vi "FPGA_AI ADC Loop.vi"(10 "AI ADC IO":T1={"AI_A"={"CONV"="RMC/DIO0", "RST"="RMC/DIO64", "SCK"="RMC/DIO17", "CS"="RMC/DIO81", "BUSY"="RMC/DIO16", "DOUT_A"="RMC/DIO48", "DOUT_B"="RMC/DIO80", "t_RST (ticks)"=0, "t_CONV (ticks)"=0, "t_BUSYMAX (ticks)"=0}, "AI_B"={"CONV"="RMC/DIO33", "RST"="RMC/DIO18", "SCK"="RMC/DIO50", "CS"="RMC/DIO32", "BUSY"="RMC/DIO65", "DOUT_A"="RMC/DIO49", "DOUT_B"="RMC/DIO82", "t_RST (ticks)"=0, "t_CONV (ticks)"=0, "t_BUSYMAX (ticks)"=0}, "AI_C"={"CONV"="RMC/DIO51", "RST"="RMC/DIO84", "SCK"="RMC/DIO2", "CS"="RMC/DIO66", "BUSY"="RMC/DIO19", "DOUT_A"="RMC/DIO83", "DOUT_B"="RMC/DIO1", "t_RST (ticks)"=0, "t_CONV (ticks)"=0, "t_BUSYMAX (ticks)"=0}}, 11 "AI ADC Loop Data In":T2={"AI ADC Loop State"=enum."Initialize", "AI Data"=[0, 0, 0, 0, 0, 0, 0, 0, 0, 0, 0, 0, 0, 0, 0, 0, 0, 0, 0, 0, 0, 0, 0, 0]}) -> (3 "AI ADC Loop Data Out":T2={"AI ADC Loop State"=enum."Initialize", "AI Data"=[0, 0, 0, 0, 0, 0, 0, 0, 0, 0, 0, 0, 0, 0, 0, 0, 0, 0, 0, 0, 0, 0, 0, 0]})   [LabVIEW 2018]
uses:
  Data Def/FPGA_AI ADC Loop Data.ctl
  Data Def/FPGA_AI ADC Loop State.ctl
  Data Def/FPGA_AI ADC IO.ctl
  24AIO/AI/AI_FPGA.lvlib
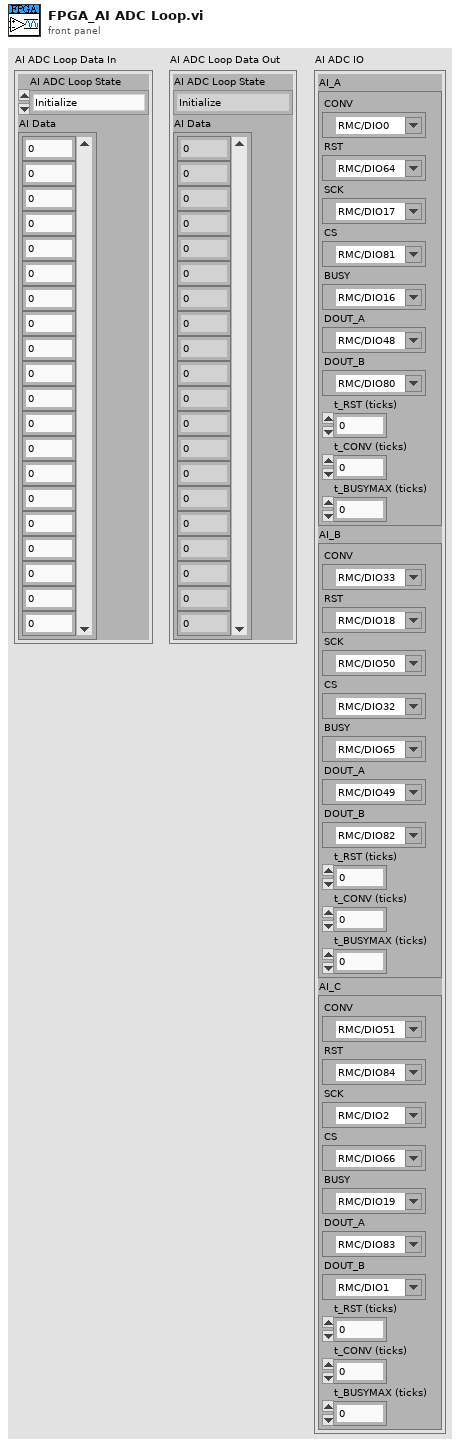
[diagram p1: front panel]
types:
  T1 = typedef "FPGA_AI ADC IO.ctl" = cluster{"AI_A":cluster{"CONV":refnum<k21>, "RST":refnum<k21>, "SCK":refnum<k21>, "CS":refnum<k21>, "BUSY":refnum<k21>, "DOUT_A":refnum<k21>, "DOUT_B":refnum<k21>, "t_RST (ticks)":u32, "t_CONV (ticks)":u32, "t_BUSYMAX (ticks)":u32}, "AI_B":cluster{"CONV":refnum<k21>, "RST":refnum<k21>, "SCK":refnum<k21>, "CS":refnum<k21>, "BUSY":refnum<k21>, "DOUT_A":refnum<k21>, "DOUT_B":refnum<k21>, "t_RST (ticks)":u32, "t_CONV (ticks)":u32, "t_BUSYMAX (ticks)":u32}, "AI_C":cluster{"CONV":refnum<k21>, "RST":refnum<k21>, "SCK":refnum<k21>, "CS":refnum<k21>, "BUSY":refnum<k21>, "DOUT_A":refnum<k21>, "DOUT_B":refnum<k21>, "t_RST (ticks)":u32, "t_CONV (ticks)":u32, "t_BUSYMAX (ticks)":u32}}
  T2 = typedef "FPGA_AI ADC Loop Data.ctl" = cluster{"AI ADC Loop State":T3, "AI Data":i16[]}
  T3 = typedef "FPGA_AI ADC Loop State.ctl" = enum16{"Initialize", "Get Data"}
  T4 = cluster{"CONV":refnum<k21>, "RST":refnum<k21>, "SCK":refnum<k21>, "CS":refnum<k21>, "BUSY":refnum<k21>, "DOUT_A":refnum<k21>, "DOUT_B":refnum<k21>, "t_RST (ticks)":u32, "t_CONV (ticks)":u32, "t_BUSYMAX (ticks)":u32}
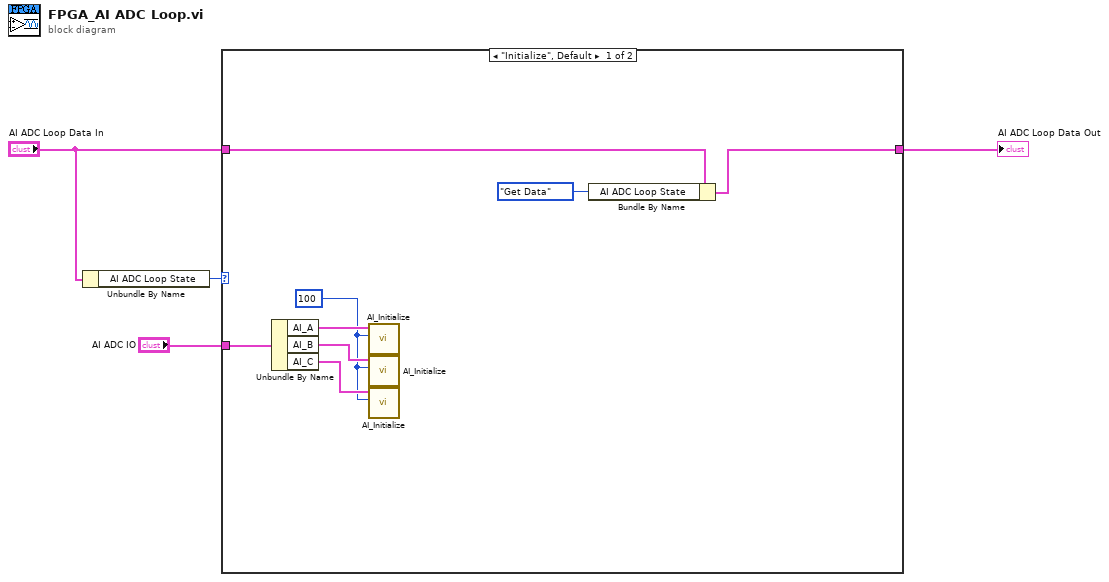
[diagram p0: block diagram]
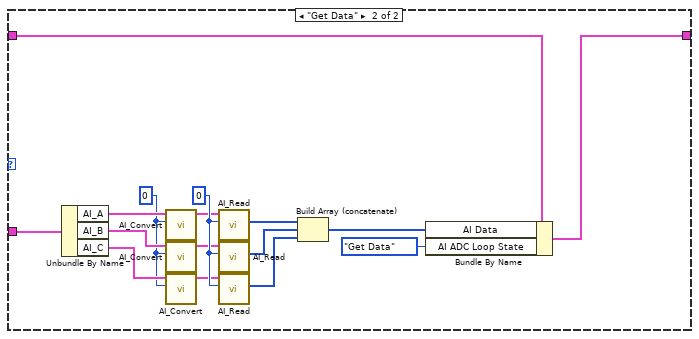
[diagram p2: hidden frame]
diagram:
  n1 = Unbundle By Name("AI ADC Loop Data In") -> ("AI ADC Loop State"=w4:T3)
  n2 = case shown="\"Initialize\", Default" w4 {
    tunnel: "AI ADC Loop Data In" -> [w11 w24]
    tunnel: [w7 w23] -> w2
    tunnel: "AI ADC IO" -> [w5 w21]
    frame "Initialize", Default {
      w8 = u32 100 ("t_RST (ticks)")
      n3 = Unbundle By Name(w5) -> ("AI_A"=w12:T4, "AI_B"=w10:T4, "AI_C"=w9:T4)
      n4 = call "AI_Initialize.vi"("t_RST (ticks)"=w8, "AD7606_IO in"=w12) -> ()  [unwired: 9 in, 1 out]
      n5 = call "AI_Initialize.vi"("t_RST (ticks)"=w8, "AD7606_IO in"=w10) -> ()  [unwired: 9 in, 1 out]
      n6 = call "AI_Initialize.vi"("t_RST (ticks)"=w8, "AD7606_IO in"=w9) -> ()  [unwired: 9 in, 1 out]
      n7 = Bundle By Name(cluster=w11, "AI ADC Loop State"=FPGA_AI_ADC_Loop_State."Get Data") -> (w7:T2)
    }
    frame "Get Data" {
      w20 = u32 0 ("t_CONV (ticks)")
      w25 = u32 0 ("t_CONV (ticks)")
      n8 = Unbundle By Name(w21) -> ("AI_A"=w28:T4, "AI_B"=w27:T4, "AI_C"=w26:T4)
      n9 = call "AI_Convert.vi"("t_CONV (ticks)"=w25, "AD7606_IO in"=w28) -> ("AD7606_IO out"=w19:T4)  [unwired: 9 in]
      n10 = call "AI_Convert.vi"("t_CONV (ticks)"=w25, "AD7606_IO in"=w27) -> ("AD7606_IO out"=w18:T4)  [unwired: 9 in]
      n11 = call "AI_Convert.vi"("t_CONV (ticks)"=w25, "AD7606_IO in"=w26) -> ("AD7606_IO out"=w17:T4)  [unwired: 9 in]
      n12 = call "AI_Read.vi"("t_CLK (ticks)"=w20, "AD7606_IO in"=w19) -> ("Data[]"=w16:i16[])  [unwired: 8 in, 1 out]
      n13 = call "AI_Read.vi"("t_CLK (ticks)"=w20, "AD7606_IO in"=w18) -> ("Data[]"=w15:i16[])  [unwired: 8 in, 1 out]
      n14 = call "AI_Read.vi"("t_CLK (ticks)"=w20, "AD7606_IO in"=w17) -> ("Data[]"=w14:i16[])  [unwired: 8 in, 1 out]
      n15 = Build Array (concatenate)(w16, w15, w14) -> (w13:i16[])
      n16 = Bundle By Name(cluster=w24, "AI Data"=w13, "AI ADC Loop State"=FPGA_AI_ADC_Loop_State."Get Data") -> (w23:T2)
    }
  }
  "AI ADC Loop Data Out" <- w2
